vi "processData.vi"(8 "error in (no error)":errorcluster, 10 "model":refnum<class "Model.lvclass">, 11 "State in":refnum<class "State.lvclass">) -> (0 "error out":errorcluster, 2 "model 2":refnum<class "Model.lvclass">, 3 "State out":refnum<class "State.lvclass">)   [LabVIEW 2013, in "State.lvclass"]
uses:
  State.lvclass
  Model/Model/Model.lvclass
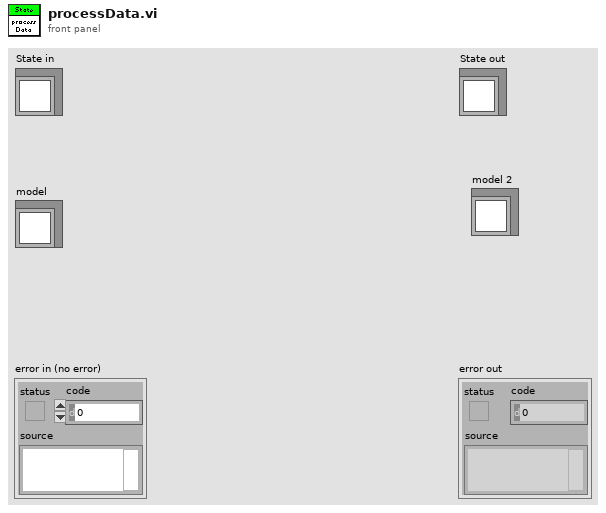
[diagram p1: front panel]
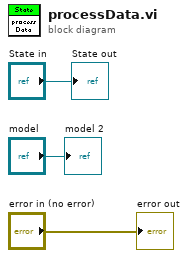
[diagram p0: block diagram]
diagram:
  "error out" <- "error in (no error)"
  "State out" <- "State in"
  "model 2" <- "model"
